vi "Requests.vi"(8 "error in (no error)":errorcluster, 9 "write enable":bool=TRUE, 11 "TEST in":refnum<class "TEST1.lvclass">) -> (0 "error out":errorcluster, 3 "TEST out":refnum<class "TEST1.lvclass">)   [LabVIEW 2021, in "TEST1.lvclass"]
uses:
  TEST1.lvclass
  D:/my_projects/projects/Algorithms/Labview/21/Master CR/Master CR.lvclass
  D:/my_projects/projects/Algorithms/Labview/21/Master CR/Devices/ET7000/TCP/TCP.lvclass
  Master CR.lvclass/Master CR.ctl
  Modbus_v121c/Modbus Data Unit/Modbus Data Unit.lvclass/Modbus Data Unit.ctl
  Modbus_v121c/Network Protocol/Network Master/Network Master.lvclass/Network Master.ctl
  Network Protocol/Read Network Protocol.vi
  Modbus_v121c/Master Function Definition/Read Discrete Inputs Request.vi
  Modbus_v121c/Network Protocol/Network Master/Read write Master.vi
  Modbus_v121c/Master Function Definition/Read Discrete Inputs Response.vi
  Modbus_v121c/Master Function Definition/Read Input Registers Request.vi
  Modbus_v121c/Master Function Definition/Read Input Registers Response.vi
  Modbus_v121c/Master Function Definition/Write Multiple Coils Request.vi
  Modbus_v121c/Master Function Definition/Function data mismatch error.vi
  Modbus_v121c/Master Function Definition/Write Multiple Coils Response.vi
  Modbus_v121c/Master Function Definition/Write Multiple Registers Request.vi
  Modbus_v121c/Master Function Definition/Write Multiple Registers Response.vi
  Modbus_v121c/Modbus Data Unit/Construct PDU.vi
  Modbus_v121c/Utility/Bytes to Bits.vi
  Modbus_v121c/Master Function Definition/Function code mismatch error.vi
  Modbus_v121c/Data Model/Error Generator.vi
  Modbus_v121c/Modbus Data Unit/Deconstruct PDU.vi
  Modbus_v121c/Utility/Bytes to U16s.vi
  Modbus_v121c/Utility/Bits to Bytes.vi
  Modbus_v121c/Utility/U16s to Bytes.vi
  TCP/TCP.lvclass
  Modbus_v121c/Network Protocol/Network Master/Network Master.lvclass
  Modbus_v121c/Modbus Data Unit/Modbus Data Unit.lvclass
  Modbus_v121c/Data Model/Device Data Model.lvclass
  Modbus_v121c/Transmission Data Unit/Transmission Data Unit.lvclass
  Master CR.lvclass
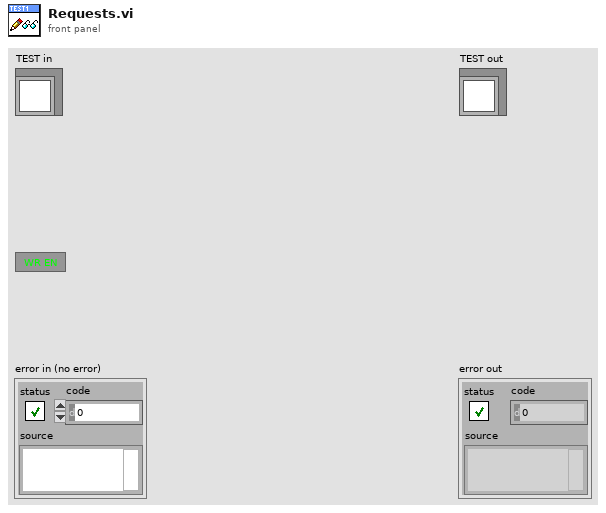
[diagram p1: front panel]
types:
  T1 = typedef "Device Data Model.lvclass/N channel.ctl" = cluster{"N DI channel":i32, "N DO channel":i32, "N AI channel":i32, "N AO channel":i32}
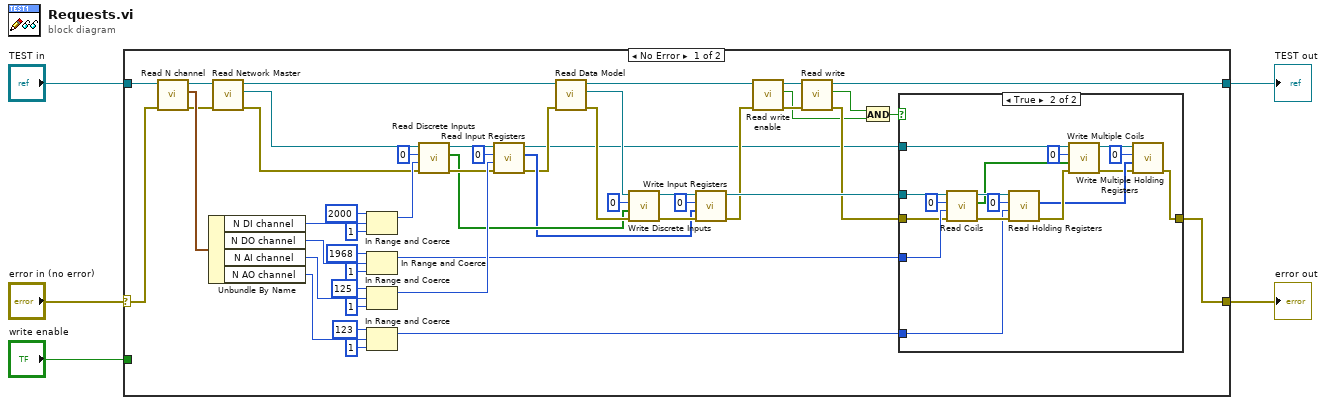
[diagram p0: block diagram]
diagram:
  n1 = case shown="No Error" "error in (no error)" {
    selector: "error in (no error)" -> [w51 w74]
    tunnel: [w21 w74] -> w3
    tunnel: [w11 w73] -> w4
    tunnel: "TEST in" -> [w52 w73]
    tunnel: "write enable" -> [_ _]
    frame No Error {
      n2 = call "Read N channel.vi"("error in (no error)"=w51, "Master CR in"=w52) -> ("error out"=w9:errorcluster, "N channel"=w53:T1, "Master CR out"=w6:refnum<class "TEST1.lvclass">)  [unwired: 7 in]
      n3 = Unbundle By Name(w53) -> ("N DI channel"=w46:i32, "N DO channel"=w33:i32, "N AI channel"=w39:i32, "N AO channel"=w36:i32)
      n4 = call "Read Network Master.vi"("error in (no error)"=w9, "TCP in"=w6) -> ("error out"=w8:errorcluster, "Network Master"=w7:refnum<class "Network Master.lvclass">, "TCP out"=w10:refnum<class "TEST1.lvclass">)  [unwired: 7 in]
      n5 = In Range and Coerce(upper limit=u16 2000, x=w46, lower limit=u16 1) -> (coerced(x)=w42:i32)  [unwired: 1 out]
      n6 = In Range and Coerce(upper limit=u16 1968, x=w33, lower limit=u16 1) -> (coerced(x)=w23:i32)  [unwired: 1 out]
      n7 = In Range and Coerce(upper limit=u16 125, x=w39, lower limit=u16 1) -> (coerced(x)=w32:i32)  [unwired: 1 out]
      n8 = In Range and Coerce(upper limit=u16 123, x=w36, lower limit=u16 1) -> (coerced(x)=w22:i32)  [unwired: 1 out]
      n9 = call "Read Discrete Inputs.vi"("error in (no error)"=w8, "number of discrete inputs"=w42, "starting address"=u16 0, "Modbus master in"=w7) -> ("error out"=w31:errorcluster, "discrete input values"=w29:bool[], "Modbus master out"=w30:refnum<class "Network Master.lvclass">)  [unwired: 5 in]
      n10 = call "Read Input Registers.vi"("error in (no error)"=w31, "number of input registers"=w32, "starting address"=u16 0, "Modbus master in"=w30) -> ("error out"=w25:errorcluster, "register values"=w26:u16[], "Modbus master out"=w12:refnum<class "Network Master.lvclass">)  [unwired: 5 in]
      n11 = call "Read Data Model.vi"("error in (no error)"=w25, "Master CR in"=w10) -> ("error out"=w49:errorcluster, "Data Model"=w48:refnum<class "Device Data Model.lvclass">, "Master CR out"=w18:refnum<class "TEST1.lvclass">)  [unwired: 7 in]
      n12 = call-dynamic "Write Discrete Inputs.vi"("error in (no error)"=w49, "input values"=w29, "starting address"=u16 0, "Device Data Model in"=w48) -> ("error out"=w27:errorcluster, "Device Data Model out"=w28:refnum<class "Device Data Model.lvclass">)  [unwired: 6 in]
      n13 = call-dynamic "Write Input Registers.vi"("error in (no error)"=w27, "register values"=w26, "starting address"=u16 0, "Device Data Model in"=w28) -> ("error out"=w19:errorcluster, "Device Data Model out"=w24:refnum<class "Device Data Model.lvclass">)  [unwired: 6 in]
      n14 = call "Read write enable.vi"("error in (no error)"=w19, "Master CR in"=w18) -> ("error out"=w16:errorcluster, "write enable"=w13:bool, "Master CR out"=w17:refnum<class "TEST1.lvclass">)  [unwired: 7 in]
      n15 = call "Read write.vi"("error in (no error)"=w16, "Master CR in"=w17) -> ("error out"=w15:errorcluster, "Write"=w14:bool, "Master CR out"=w11:refnum<class "TEST1.lvclass">)  [unwired: 7 in]
      n16 = And(x=w14, y=w13) -> (x .and. y?=w20:bool)
      n17 = case shown="True" w20 {
        tunnel: w24 -> [_ w72]
        tunnel: w23 -> [_ w67]
        tunnel: w22 -> [_ w66]
        tunnel: [w55 w58] -> w21
        tunnel: w15 -> [w55 w57]
        tunnel: w12 -> [_ w56]
        frame False {
        }
        frame True {
          n18 = call-dynamic "Read Coils.vi"("error in"=w57, "number of coils"=w67, "starting address"=u16 0, "device data model in"=w72) -> ("error out"=w70:errorcluster, "data"=w64:bool[], "device data model out"=w71:refnum<class "Device Data Model.lvclass">)  [unwired: 5 in]
          n19 = call-dynamic "Read Holding Registers.vi"("error in"=w70, "number of registers"=w66, "starting address"=u16 0, "device data model in"=w71) -> ("error out"=w65:errorcluster, "data"=w60:u16[])  [unwired: 5 in, 1 out]
          n20 = call "Write Multiple Coils.vi"("error in (no error)"=w65, "coil values"=w64, "starting address"=u16 0, "Modbus master in"=w56) -> ("error out"=w59:errorcluster, "Modbus master out"=w62:refnum<class "Network Master.lvclass">)  [unwired: 6 in]
          n21 = call "Write Multiple Holding Registers.vi"("error in (no error)"=w59, "holding register values"=w60, "starting address"=u16 0, "Modbus master in"=w62) -> ("error out"=w58:errorcluster)  [unwired: 6 in, 1 out]
        }
      }
    }
    frame Error {
    }
  }
  "error out" <- w3
  "TEST out" <- w4
